vi "TetroStateChecker.vi"(8 "Tetro Info":T1) -> (2 "isNewTetro":bool)   [LabVIEW 2026]
doc: "This Logic VI checks, whether a new tetromino needs to be inserted or another one is still actively falling."
uses:
  02_StateMachine/GameTetrominoInformationTypeDef.ctl
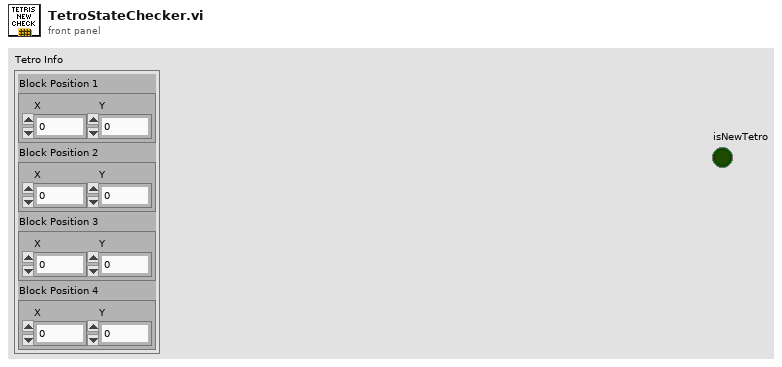
[diagram p1: front panel]
types:
  T1 = typedef "GameTetrominoInformationTypeDef.ctl" = cluster{"Block Position 1":cluster{"X":i32, "Y":i32}, "Block Position 2":cluster{"X":i32, "Y":i32}, "Block Position 3":cluster{"X":i32, "Y":i32}, "Block Position 4":cluster{"X":i32, "Y":i32}}
  T2 = cluster{"Block Position 1":cluster{"X":bool, "Y":bool}, "Block Position 2":cluster{"X":bool, "Y":bool}, "Block Position 3":cluster{"X":bool, "Y":bool}, "Block Position 4":cluster{"X":bool, "Y":bool}}
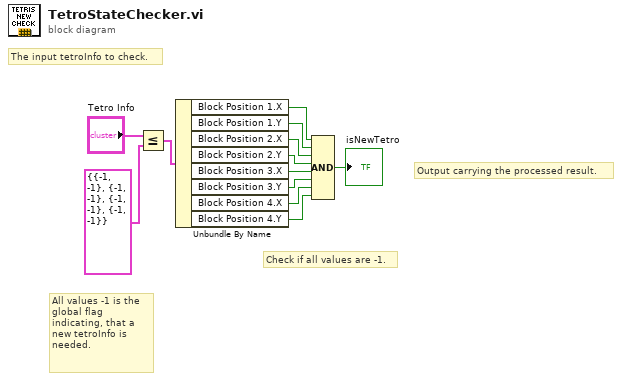
[diagram p0: block diagram]
diagram:
  # "Output carrying the processed result."
  # "The input tetroInfo to check."
  # "Check if all values are -1."
  # "All values -1 is the global flag indicating, that a new tetroInfo is needed."
  n1 = Less Or Equal?(x="Tetro Info", y=T1 {"Block Position 1"={"X"=-1, "Y"=-1}, "Block Position 2"={"X"=-1, "Y"=-1}, "Block Position 3"={"X"=-1, "Y"=-1}, "Block Position 4"={"X"=-1, "Y"=-1}}) -> (x <= y?=w10:T2)
  n2 = Unbundle By Name(w10) -> ("Block Position 1.X"=w9:bool, "Block Position 1.Y"=w8:bool, "Block Position 2.X"=w7:bool, "Block Position 2.Y"=w6:bool, "Block Position 3.X"=w5:bool, "Block Position 3.Y"=w4:bool, "Block Position 4.X"=w3:bool, "Block Position 4.Y"=w2:bool)
  n3 = Compound Arithmetic op=AND(w9, w8, w7, w6, w5, w4, w3, w2) -> (→"isNewTetro":bool)
